vi "Pins to Set.vi"(11 "pin or relay names array":string[](array[string])) -> (3 "pin or relay name set":set{string}(c389))   [LabVIEW 2020, in "Measurement Plugin Session Management V1.lvlib" / "Session Reservation.lvclass"]
uses:
  Session Reservation.lvclass
  Session Reservation.lvclass/Session Reservation.ctl
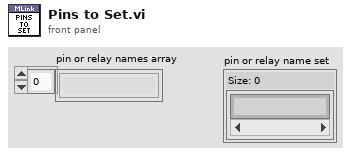
[diagram p1: front panel]
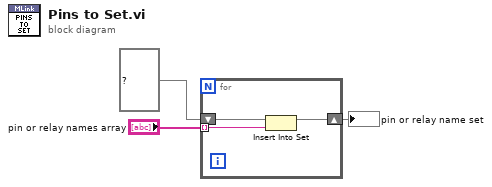
[diagram p0: block diagram]
diagram:
  n1 = for {
    tunnel: "pin or relay names array" -> [w4] mode=indexing
    shift-right: [w5] -> w1
    shift-left: set{string} {} ("pin or relay name set") -> [w6]
    n2 = Insert Into Set(10:w4, 11:w6) -> (3:w5:set{string})  [unwired: 1 out]
  }
  "pin or relay name set" <- w1
